vi "Debug Read All.vi"(8 "error in (no error)":errorcluster, 11 "TD4 in":refnum<class "TD4.lvclass">) -> (0 "error out":errorcluster, 2 "Debug Output":T1, 3 "TD4 out":refnum<class "TD4.lvclass">)   [LabVIEW 2025, in "TD4.lvclass"]
uses:
  TD4.lvclass
  TD4.lvclass/TD4.ctl
  Debug Output.ctl
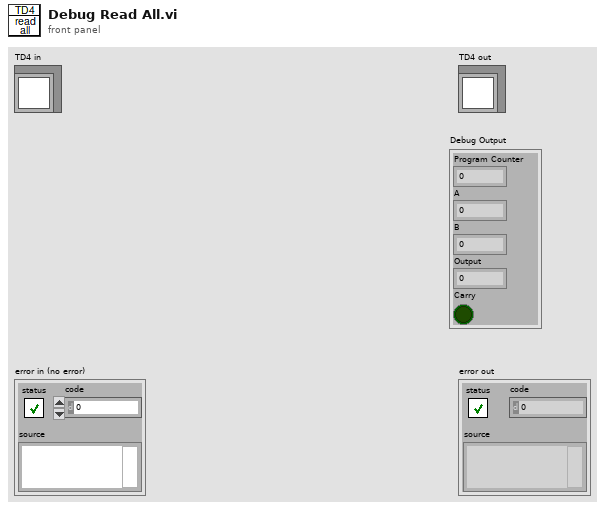
[diagram p1: front panel]
types:
  T1 = typedef "TD4.lvclass/Debug Output.ctl" = cluster{"Program Counter":u8, "A":u8, "B":u8, "Output":u8, "Carry":bool}
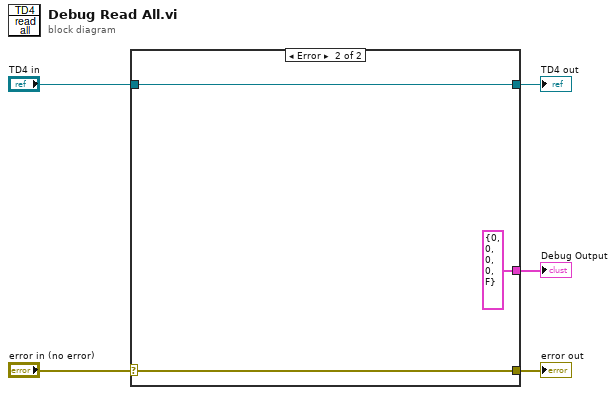
[diagram p0: block diagram]
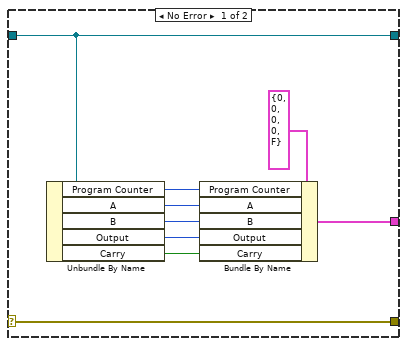
[diagram p2: hidden frame]
diagram:
  n1 = case shown="Error" "error in (no error)" {
    selector: "error in (no error)" -> [w14 w16]
    tunnel: [w14 w16] -> w4
    tunnel: [w13 w17] -> w2
    tunnel: "TD4 in" -> [w13 w17]
    tunnel: [w6 T1 {"Program Counter"=0, "A"=0, "B"=0, "Output"=0, "Carry"=FALSE} ("Debug Output 2")] -> w1
    frame No Error {
      n2 = Unbundle By Name(w13) -> ("Program Counter"=w12:u8, "A"=w11:u8, "B"=w10:u8, "Output"=w9:u8, "Carry"=w8:bool)
      n3 = Bundle By Name(cluster=T1 {"Program Counter"=0, "A"=0, "B"=0, "Output"=0, "Carry"=FALSE} ("Debug Output 2"), "Program Counter"=w12, "A"=w11, "B"=w10, "Output"=w9, "Carry"=w8) -> (w6:T1)
    }
    frame Error {
    }
  }
  "error out" <- w4
  "TD4 out" <- w2
  "Debug Output" <- w1
